vi "ExtractValues.vi"(1 "Variable name":string, 2 "Input String":string) -> (0 "Variable value":dbl)   [LabVIEW 2018]
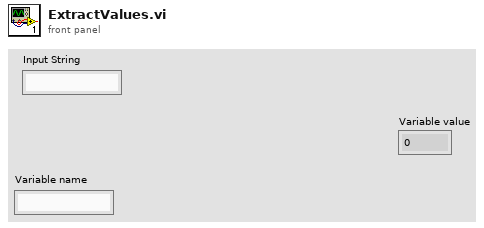
[diagram p1: front panel]
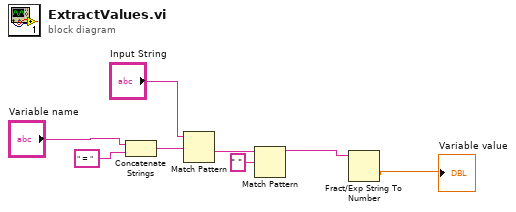
[diagram p0: block diagram]
diagram:
  n1 = Concatenate Strings("Variable name", " = " ("string")) -> (w6:string)
  n2 = Match Pattern(string="Input String", regular expression=w6) -> (after substring=w4:string)  [unwired: 1 in, 3 out]
  n3 = Match Pattern(string=w4, regular expression=" ") -> (before substring=w2:string)  [unwired: 1 in, 3 out]
  n4 = Fract/Exp String To Number(string=w2) -> (number=→"Variable value":dbl)  [unwired: 3 in, 1 out]
